vi "PumpVol.vi"(8 "error in (no error)":errorcluster, 10 "volume to pump":dbl, 11 "SimPump in":refnum<class "SimPump.lvclass">) -> (0 "error out":errorcluster, 3 "SimPump out":refnum<class "SimPump.lvclass">)   [LabVIEW 2019, in "SimPump.lvclass"]
doc: "Commands the pump to pump the requested volume.\n\nwww.sciware.com.au"
uses:
  SimPump.lvclass
  Private/CmdQueueType.ctl
  SimPump.lvclass/SimPump.ctl
panel:
  # "BSD License (http://www.opensource.org/licenses/bsd-license.php)"
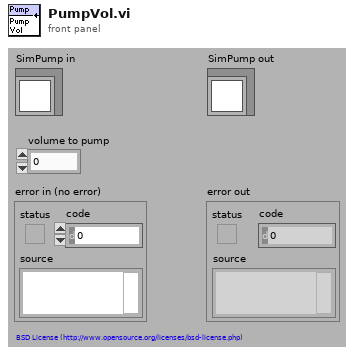
[diagram p1: front panel]
types:
  T1 = typedef "SimPump.lvclass/CmdQueueType.ctl" = string
  T2 = typedef "SimPump.lvclass/CmdQueueRef.ctl" = refnum<queue>
  T3 = typedef "SimPump.lvclass/DataRef.ctl" = refnum<data-value>
  T4 = typedef "SimPump.lvclass/DataMembers.ctl" = cluster{"flow rate":dbl, "volume to pump":dbl, "state":bool, "ti":u32, "t0":u32}
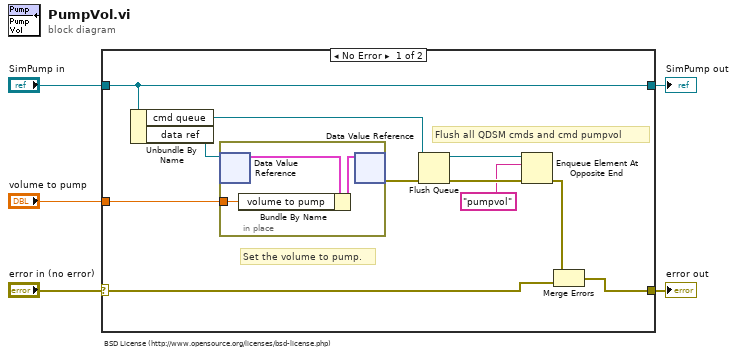
[diagram p0: block diagram]
diagram:
  # "BSD License (http://www.opensource.org/licenses/bsd-license.php)"
  n1 = case shown="No Error" "error in (no error)" {
    selector: "error in (no error)" -> [w9 w21]
    tunnel: [w8 w21] -> w4
    tunnel: [w11 w20] -> w2
    tunnel: "SimPump in" -> [w11 w20]
    tunnel: "volume to pump" -> [w7 _]
    frame No Error {
      # "Flush all QDSM cmds and cmd pumpvol"
      # "Set the volume to pump."
      n2 = Unbundle By Name(w11) -> ("cmd queue"=w10:T2, "data ref"=w16:T3)
      n3 = in-place {
        in-place-border: w7 -> [w17]
        n4 = in-place-dvr #1(w16) -> (w19:T4)  [unwired: 1 out]
        n5 = Bundle By Name(cluster=w19, "volume to pump"=w17) -> (w18:T4)
        n6 = in-place-dvr #1(w18) -> (w13:errorcluster)  [unwired: 1 out]
      }
      n7 = Flush Queue(queue=w10, error in (no error)=w13) -> (queue out=w14:T2, error out=w15:errorcluster)  [unwired: 1 out]
      n8 = Enqueue Element At Opposite End(queue=w14, element=T1 "pumpvol", error in (no error)=w15) -> (error out=w12:errorcluster)  [unwired: 1 in, 2 out]
      n9 = Merge Errors(w12, w9) -> (w8:errorcluster)
    }
    frame Error {
    }
  }
  "error out" <- w4
  "SimPump out" <- w2
